vi "Save New VI From XML.vi"(7 "Use VTT?":bool, 8 "error in (no error)":errorcluster, 9 "Block Diagram XML/VTT":string, 10 "Front Panel XML/VTT":string, 11 "Resources":T1) -> (0 "error out":errorcluster, 3 "Unique Temporary File Path":path)   [LabVIEW 2023]
uses:
  Resource Manipulation.lvlib
  Resource Manipulation/Find Resource by Type (String).vi
  Resource Manipulation/Resource.ctl
  Resource Manipulation/Resource Array.ctl
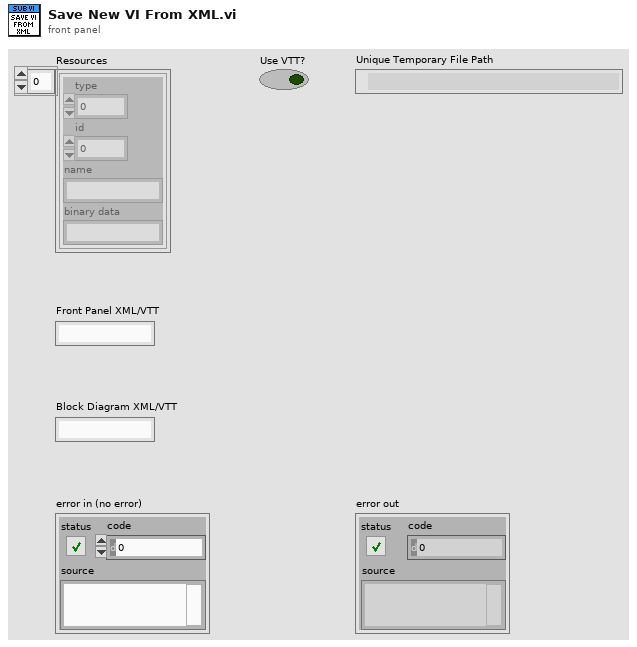
[diagram p1: front panel]
types:
  T1 = typedef "Resource Manipulation.lvlib/Resource Array.ctl" = T2[]
  T2 = typedef "Resource Manipulation.lvlib/Resource.ctl" = cluster{"type":u32, "id":i32, "name":string, "binary data":string}
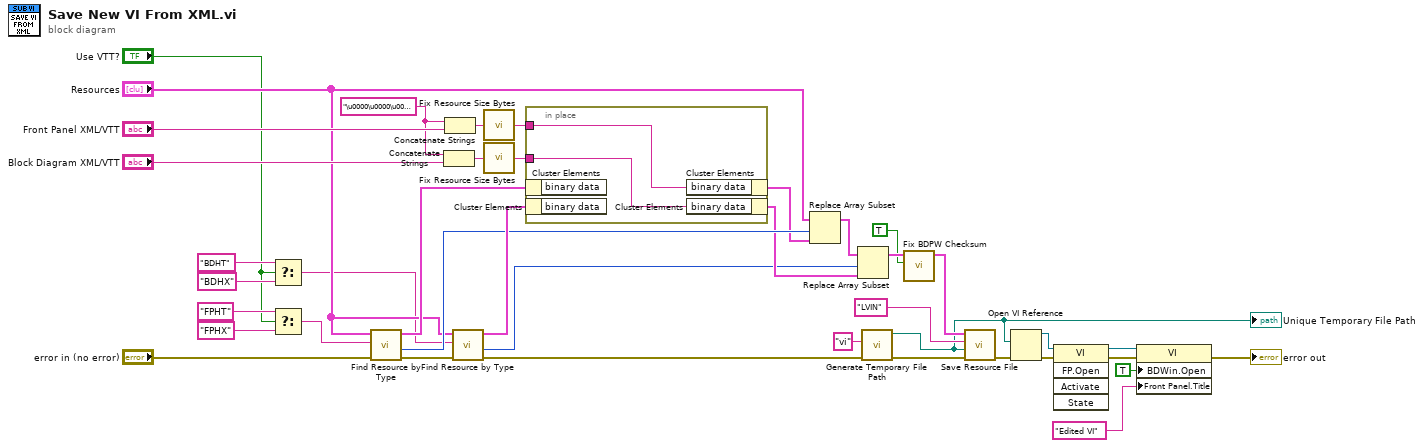
[diagram p0: block diagram]
diagram:
  w38 = "\u0000\u0000\u0000\u0000"
  n1 = Select(t="BDHT", s="Use VTT?", f="BDHX") -> (s? t:f=w2:string)
  n2 = Select(t="FPHT", s="Use VTT?", f="FPHX") -> (s? t:f=w10:string)
  n3 = call-poly "Find Resource by Type.vi"("error in (no error)"="error in (no error)", "Resource Type"=w10, "Resources"="Resources") -> ("error out"=w5:errorcluster, "Index"=w31:i32, "Resource"=w33:T2)  [unwired: 5 in, 1 out]
  n4 = Concatenate Strings(w38, "Block Diagram XML/VTT") -> (w36:string)
  n5 = Concatenate Strings(w38, "Front Panel XML/VTT") -> (w37:string)
  n6 = call-poly "Find Resource by Type.vi"("error in (no error)"=w5, "Resource Type"=w2, "Resources"="Resources") -> ("error out"=w6:errorcluster, "Index"=w28:i32, "Resource"=w32:T2)  [unwired: 5 in, 1 out]
  n7 = call "Fix Resource Size Bytes.vi"("Data in"=w37) -> ("Data out"=w35:string)
  n8 = call "Fix Resource Size Bytes.vi"("Data in"=w36) -> ("Data out"=w34:string)
  n9 = in-place {
    in-place-border: w35 -> [w42]
    in-place-border: w34 -> [w41]
    n10 = in-place-cluster #1(w33) -> ()  [unwired: 1 out]
    n11 = in-place-cluster #2(w32) -> ()  [unwired: 1 out]
    n12 = in-place-cluster #1("binary data"=w42) -> (w30:T2)
    n13 = in-place-cluster #2("binary data"=w41) -> (w29:T2)
  }
  n14 = Replace Array Subset(array="Resources", new element=w30, index=w31) -> (w27:T1)
  n15 = Replace Array Subset(array=w27, new element=w29, index=w28) -> (w20:T1)
  n16 = call <vilib>:"Generate Temporary File Path.vi"("error in (no error)"=w6, "Temporary File Extension (tmp)"="vi") -> ("error out"=w8:errorcluster, "Unique Temporary File Path"=w7:path)  [unwired: 8 in]
  "Unique Temporary File Path" <- w7
  n17 = call "Fix BDPW Checksum.vi"("Only fix 3rd hash (F)"=TRUE, "Resources in"=w20) -> ("Resources out"=w19:T1)  [unwired: 9 in]
  n18 = call "Save Resource File.vi"("error in (no error)"=w8, "Path"=w7, "File type"="LVIN", "Resources"=w19) -> ("error out"=w25:errorcluster)  [unwired: 7 in]
  n19 = Open VI Reference(vi path=w7, error in (no error)=w25) -> (vi reference=w21:refnum<vi>, error out=w17:errorcluster)  [unwired: 4 in]
  n20 = invoke class="VI" method="FP.Open"(reference=w21, error in=w17) -> (reference out=w22:refnum<vi>, error out=w16:errorcluster)  [unwired: 3 in, 3 out]
  n21 = property class="VI"(reference=w22, error in=w16, "BDWin.Open"=TRUE ("Block Diagram Window:Open"), "Front Panel.Title"="Edited VI") -> (error out=→"error out":errorcluster)  [unwired: 1 out]
